vi "Source Voltage No Meas.vi"(7 "Channel Lists":string[](array[string]), 8 "error in (no error)":errorcluster, 10 "voltage level":dbl format="%_6p", 11 "Instrument Sessions In":refnum<k15>[](array[refnum])) -> (0 "error out":errorcluster, 3 "Instrument Sessions Out":refnum<k15>[](array[refnum]))   [LabVIEW 2013]
uses:
  <instrlib>/niDCPower/nidcpower.llb/niDCPower Wait For Event - Event.ctl
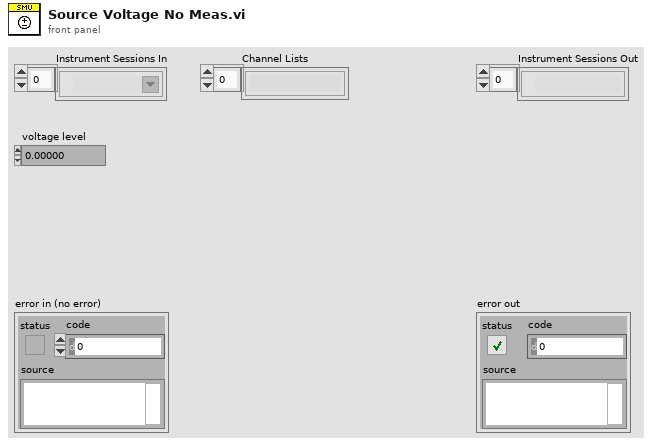
[diagram p1: front panel]
types:
  T1 = typedef "niDCPower Wait For Event - Event.ctl" = i32
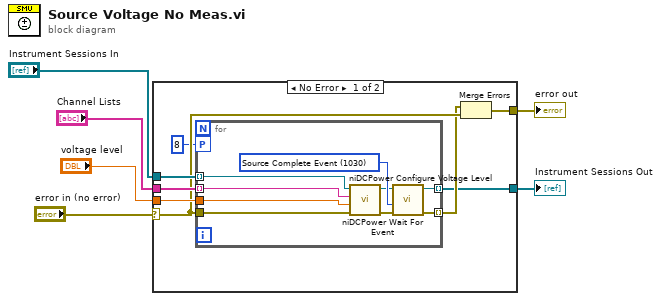
[diagram p0: block diagram]
diagram:
  n1 = case shown="No Error" "error in (no error)" {
    selector: "error in (no error)" -> [w10 w24]
    tunnel: [w14 w24] -> w6
    tunnel: "Instrument Sessions In" -> [w13 w25]
    tunnel: "Channel Lists" -> [w12 _]
    tunnel: [w7 w25] -> w3
    tunnel: "voltage level" -> [w11 _]
    frame No Error {
      n2 = for {
        tunnel: w13 -> [w23] mode=indexing
        tunnel: w12 -> [w17] mode=indexing
        tunnel: w11 -> [w22]
        tunnel: w10 -> [w21]
        workers-P: 8 -> [_]
        tunnel: [w16] -> w8 mode=indexing
        tunnel: [w15] -> w7 mode=indexing
        w19 = T1 1030 items=["Source Complete Event"=1030, "Measure Complete Event"=1031, "Sequence Iteration Complete Event"=1032, "Sequence Engine Done Event"=1033, "Pulse Complete Event"=1051, "Ready For Pulse Trigger Event"=1052] ("event")
        n3 = call <instrlib>:"niDCPower Configure Voltage Level.vi"("error in (no error)"=w21, "voltage level"=w22, "channel name"=w17, "instrument handle"=w23) -> ("error out"=w20:errorcluster, "instrument handle out"=w18:refnum<k15>)  [unwired: 6 in]
        n4 = call <instrlib>:"niDCPower Wait For Event.vi"("error in (no error)"=w20, "event"=w19, "instrument handle"=w18) -> ("error out"=w16:errorcluster, "instrument handle out"=w15:refnum<k15>)  [unwired: 7 in]
      }
      n5 = Merge Errors(w8, w10) -> (w14:errorcluster)
    }
    frame Error {
    }
  }
  "Instrument Sessions Out" <- w3
  "error out" <- w6
